vi "Operate Elevator.vi"(8 "error in (no error)":errorcluster, 10 "Joystick State":T1, 11 "Operator in":refnum<class "Operator.lvclass">) -> (0 "error out":errorcluster, 3 "Operator out":refnum<class "Operator.lvclass">)   [LabVIEW 2014, in "Operator.lvlib" / "Operator.lvclass"]
uses:
  Operator.lvclass
  Joystick/Joystick Class/Joystick State.ctl
  Joystick/Joystick Class/Button State.ctl
  Joystick/Joystick Class/Axis State.ctl
  Operator.lvclass/Operator.ctl
  Elevator/Elevator Messages/Set Rate (Percent) Msg/Set Rate (Percent) Msg.lvclass/Set Rate (Percent) Msg.ctl
  <vilib>/ActorFramework/Message Enqueuer/Message Enqueuer.lvclass/Message Enqueuer.ctl
  <vilib>/ActorFramework/Message Enqueuer/Enqueue.vi
  <vilib>/ActorFramework/Message Priority Queue/Priority Enqueue.vi
  Elevator/Elevator Messages/Set Rate (Percent) Msg/Set Rate (Percent) Msg.lvclass
  Joystick/Joystick Class/Joystick.lvclass
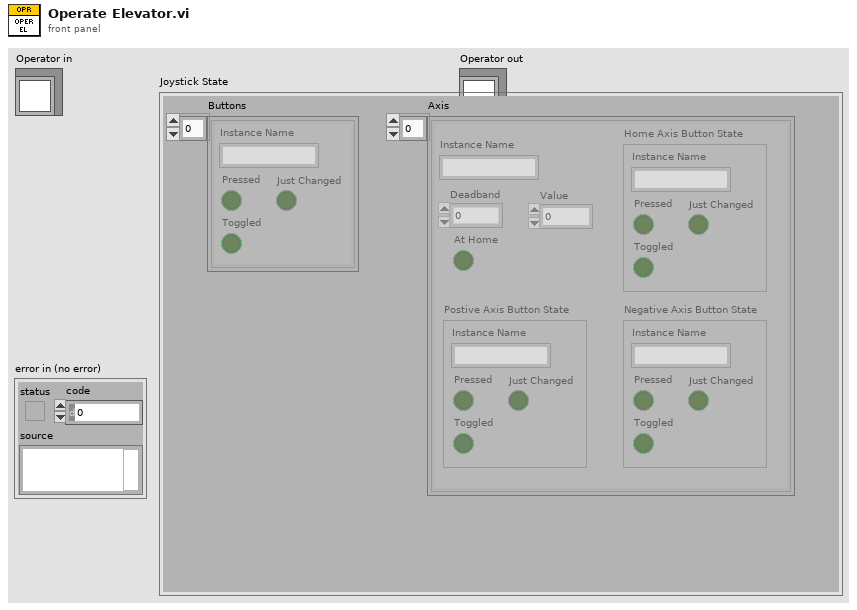
[diagram p1: front panel]
types:
  T1 = typedef "Joystick.lvlib/Joystick.lvclass/Joystick State.ctl" = cluster{"Buttons":T2[], "Axis":T3[]}
  T2 = typedef "Joystick.lvlib/Joystick.lvclass/Button State.ctl" = cluster{"Pressed":bool, "Instance Name":string, "Toggled":bool, "Just Changed":bool}
  T3 = typedef "Joystick.lvlib/Joystick.lvclass/Axis State.ctl" = cluster{"Instance Name":string, "Deadband":dbl, "Value":dbl, "At Home":bool, "Postive Axis Button State":T2, "Negative Axis Button State":T2, "Home Axis Button State":T2}
  T4 = enum16{"Critical", "Error", "Warning", "Informational", "Debug"}
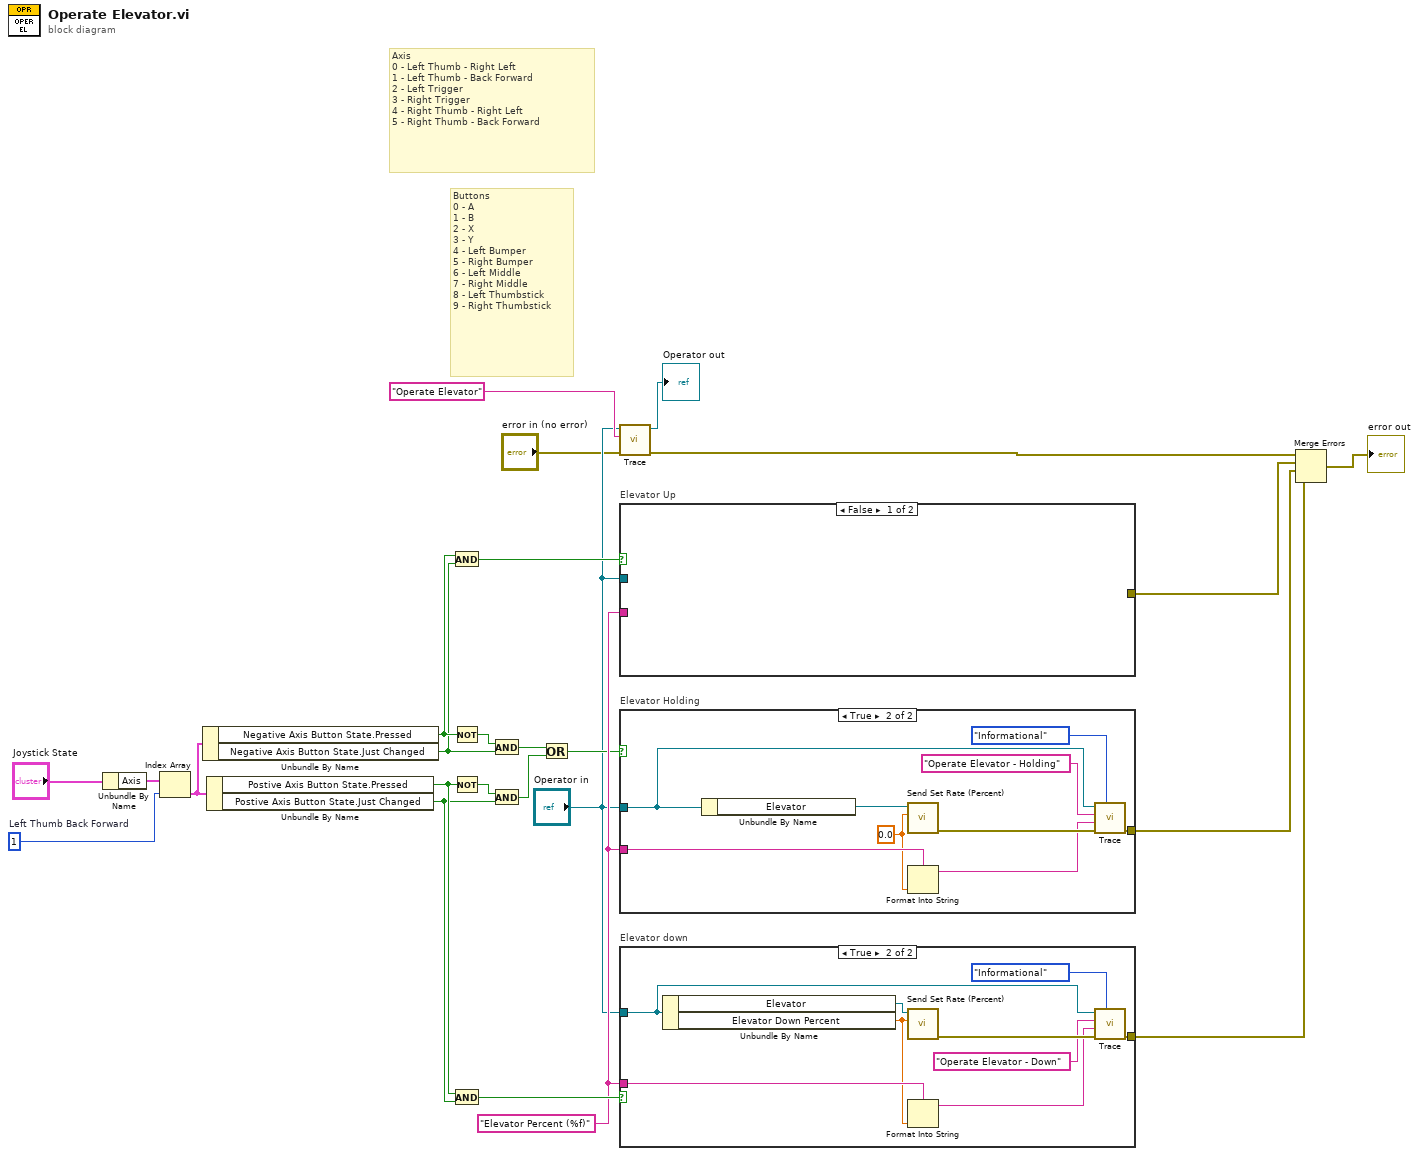
[diagram p0: block diagram]
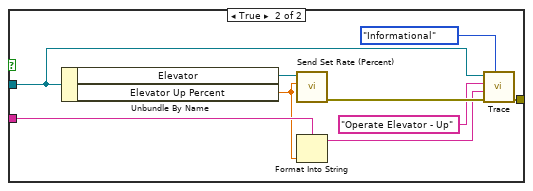
[diagram p4: hidden frame]
diagram:
  w16 = "Elevator Percent (%f)" ("format string")
  w21 = 1  # Left Thumb Back Forward
  # "Buttons\n0 - A\n1 - B\n2 - X\n3 - Y\n4 - Left Bumper\n5 - Right Bumper\n6 - Left Middle\n7 - Right Middle\n8 - Left Thumbstick\n9 - Right Thumbstick"
  # "Axis\n0 - Left Thumb - Right Left\n1 - Left Thumb - Back Forward\n2 - Left Trigger\n3 - Right Trigger\n4 - Right Thumb - Right Left\n5 - Right Thumb - Back Forward"
  n1 = Unbundle By Name("Joystick State") -> ("Axis"=w22:T3[])
  n2 = Index Array(array=w22, index=w21) -> (element=w19:T3)
  n3 = Unbundle By Name(w19) -> ("Negative Axis Button State.Pressed"=w12:bool, "Negative Axis Button State.Just Changed"=w10:bool)
  n4 = Unbundle By Name(w19) -> ("Postive Axis Button State.Pressed"=w9:bool, "Postive Axis Button State.Just Changed"=w7:bool)
  n5 = And(x=w12, y=w10) -> (x .and. y?=w18:bool)
  n6 = Not(x=w12) -> (.not. x?=w11:bool)
  n7 = Not(x=w9) -> (.not. x?=w8:bool)
  n8 = And(x=w9, y=w7) -> (x .and. y?=w17:bool)
  n9 = And(x=w11, y=w10) -> (x .and. y?=w15:bool)
  n10 = And(x=w8, y=w7) -> (x .and. y?=w14:bool)
  n11 = Or(x=w15, y=w14) -> (x .or. y?=w13:bool)
  n12 = call-dynamic "Trace.vi"("error in (no error)"="error in (no error)", "System Action"="Operate Elevator", "System Actor in"="Operator in") -> ("error out"=w23:errorcluster, "System Actor out"=→"Operator out":refnum<class "Operator.lvclass">)  [unwired: 7 in]
  n13 = case "Elevator Up" shown="False" w18 {
    tunnel: "Operator in" -> [_ w33]
    tunnel: w16 -> [_ w30]
    tunnel: [_ w26] -> w3
    frame False {
    }
    frame True {
      n14 = Unbundle By Name(w33) -> ("Elevator"=w34:refnum<class "Message Enqueuer.lvclass">, "Elevator Up Percent"=w28:dbl)
      n15 = call "Send Set Rate (Percent).vi"("Percent"=w28, "Message Enqueuer"=w34) -> ("error out"=w32:errorcluster)  [unwired: 8 in, 1 out]
      n16 = Format Into String(format string=w30, w28) -> (resulting string=w29:string)  [unwired: 2 in, 1 out]
      n17 = call-dynamic "Trace.vi"("Trace Level"=T4."Informational", "error in (no error)"=w32, "System Message"=w29, "System Action"="Operate Elevator - Up", "System Actor in"=w33) -> ("error out"=w26:errorcluster)  [unwired: 5 in, 1 out]
    }
  }
  n18 = case "Elevator Holding" shown="True" w13 {
    tunnel: "Operator in" -> [_ w42]
    tunnel: w16 -> [_ w39]
    tunnel: [_ w35] -> w2
    frame False {
    }
    frame True {
      w36 = 0.0 ("Percent")
      n19 = Unbundle By Name(w42) -> ("Elevator"=w43:refnum<class "Message Enqueuer.lvclass">)
      n20 = call "Send Set Rate (Percent).vi"("Percent"=w36, "Message Enqueuer"=w43) -> ("error out"=w41:errorcluster)  [unwired: 8 in, 1 out]
      n21 = Format Into String(format string=w39, w36) -> (resulting string=w38:string)  [unwired: 2 in, 1 out]
      n22 = call-dynamic "Trace.vi"("Trace Level"=T4."Informational", "error in (no error)"=w41, "System Message"=w38, "System Action"="Operate Elevator - Holding", "System Actor in"=w42) -> ("error out"=w35:errorcluster)  [unwired: 5 in, 1 out]
    }
  }
  n23 = case "Elevator down" shown="True" w17 {
    tunnel: "Operator in" -> [_ w51]
    tunnel: w16 -> [_ w48]
    tunnel: [_ w44] -> w1
    frame False {
    }
    frame True {
      n24 = Unbundle By Name(w51) -> ("Elevator"=w52:refnum<class "Message Enqueuer.lvclass">, "Elevator Down Percent"=w46:dbl)
      n25 = call "Send Set Rate (Percent).vi"("Percent"=w46, "Message Enqueuer"=w52) -> ("error out"=w50:errorcluster)  [unwired: 8 in, 1 out]
      n26 = Format Into String(format string=w48, w46) -> (resulting string=w47:string)  [unwired: 2 in, 1 out]
      n27 = call-dynamic "Trace.vi"("Trace Level"=T4."Informational", "error in (no error)"=w50, "System Message"=w47, "System Action"="Operate Elevator - Down", "System Actor in"=w51) -> ("error out"=w44:errorcluster)  [unwired: 5 in, 1 out]
    }
  }
  n28 = Merge Errors(w23, w3, w2, w1) -> (→"error out":errorcluster)
